vi "Read_serverTimeout.vi"(8 "error in (no error)":errorcluster, 11 "TcpServerBase in":refnum<class "TcpServerBase.lvclass">) -> (0 "error out":errorcluster, 2 "serverTimeout":i32, 3 "TcpServerBase out":refnum<class "TcpServerBase.lvclass">)   [LabVIEW 2018, in "TcpServerBase.lvclass"]
doc: "Read timeout server."
uses:
  TcpServerBase.lvclass
  TcpServerBase.lvclass/TcpServerBase.ctl
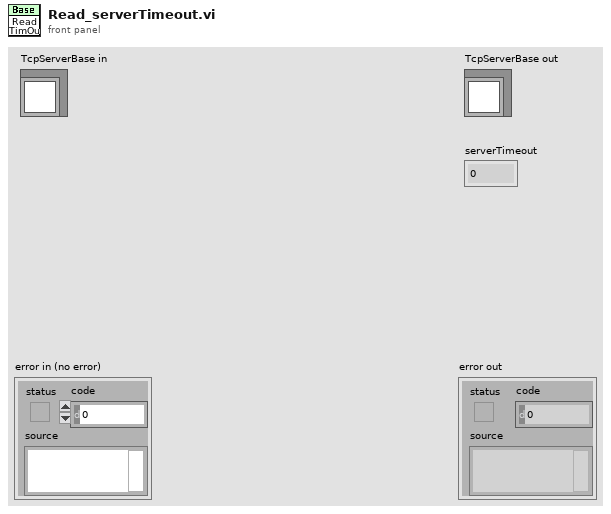
[diagram p1: front panel]
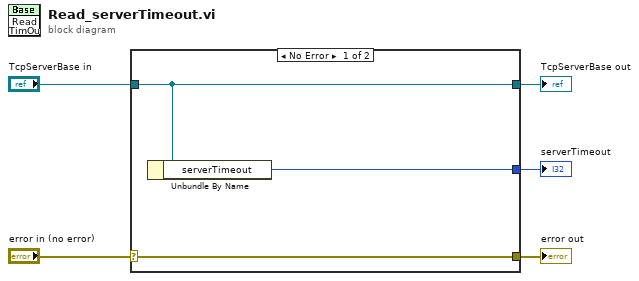
[diagram p0: block diagram]
diagram:
  n1 = case shown="No Error" "error in (no error)" {
    selector: "error in (no error)" -> [w8 w9]
    tunnel: [w8 w9] -> w4
    tunnel: [w7 w10] -> w2
    tunnel: "TcpServerBase in" -> [w7 w10]
    tunnel: [w6 _] -> w1
    frame No Error {
      n2 = Unbundle By Name(w7) -> ("serverTimeout"=w6:i32)
    }
    frame Error {
    }
  }
  "error out" <- w4
  "TcpServerBase out" <- w2
  "serverTimeout" <- w1
